vi "CLI_GetParamValue.vi"(8 "error in (no error)":errorcluster caption="entrée d'erreur (pas d'erreur)", 10 "ParsedParameters":cluster{"Name":string, "Value":string}[](array[cluster]), 11 "SearchParam":string) -> (0 "Error out":errorcluster, 2 "Exist":bool, 3 "ParamValue":string)   [LabVIEW 2013]
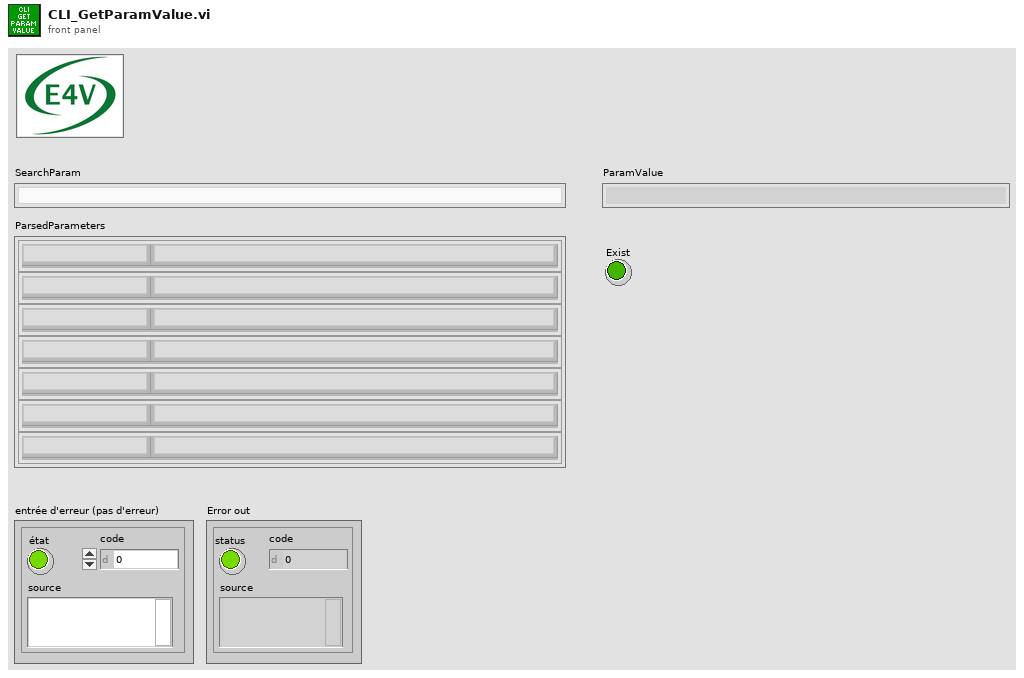
[diagram p1: front panel]
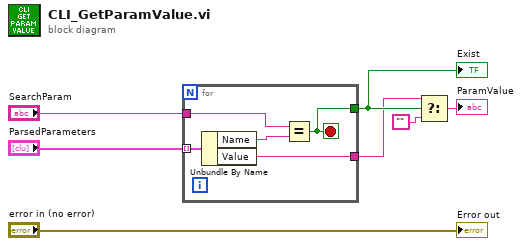
[diagram p0: block diagram]
diagram:
  n1 = for {
    tunnel: "ParsedParameters" -> [w11] mode=indexing
    tunnel: "SearchParam" -> [w12]
    tunnel: [w9] -> w2
    tunnel: [w8] -> w4
    stop <- w8 stop-if-true
    n2 = Unbundle By Name(w11) -> ("Name"=w10:string, "Value"=w9:string)
    n3 = Equal?(x=w12, y=w10) -> (x = y?=w8:bool)
  }
  "Exist" <- w4
  n4 = Select(t=w2, s=w4, f="") -> (s? t:f=→"ParamValue":string)
  "Error out" <- "error in (no error)"
